vi "FT10_Log Tester Write TDMS.vi"(6 "Time in":timestamp, 8 "error in (no error)":errorcluster, 9 "Measurements in":T1, 10 "Waveform in":waveform(dbl), 11 "Refnum in":refnum<k34>) -> (0 "error out":errorcluster, 3 "Refnum out":refnum<k34>)   [LabVIEW 2015]
uses:
  <vilib>/Waveform/WDTOps.llb/WDT Number of Waveform Samples DBL.vi
  <vilib>/Waveform/WDTOps.llb/WDT Get Waveform Time Array DBL.vi
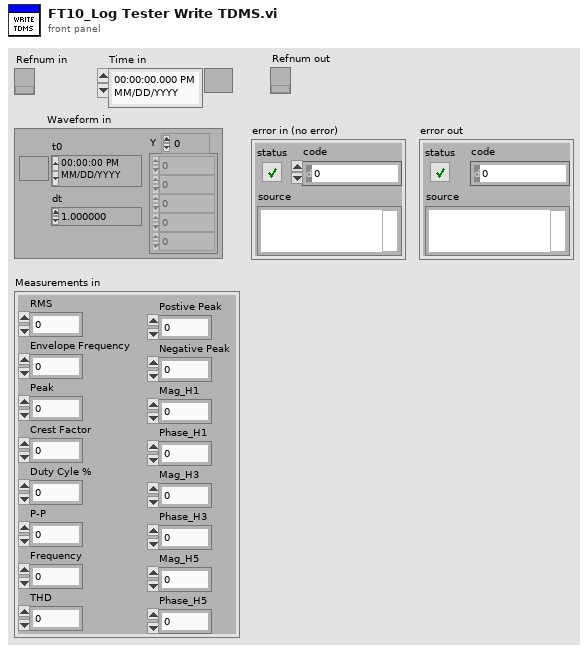
[diagram p1: front panel]
types:
  T1 = cluster{"RMS":dbl, "Envelope Frequency":dbl, "Peak":dbl, "Crest Factor":dbl, "Duty Cyle %":dbl, "P-P":dbl, "Frequency":dbl, "THD":dbl, "Postive Peak":dbl, "Negative Peak":dbl, "Mag_H1":dbl, "Phase_H1":dbl, "Mag_H3":dbl, "Phase_H3":dbl, "Mag_H5":dbl, "Phase_H5":dbl}
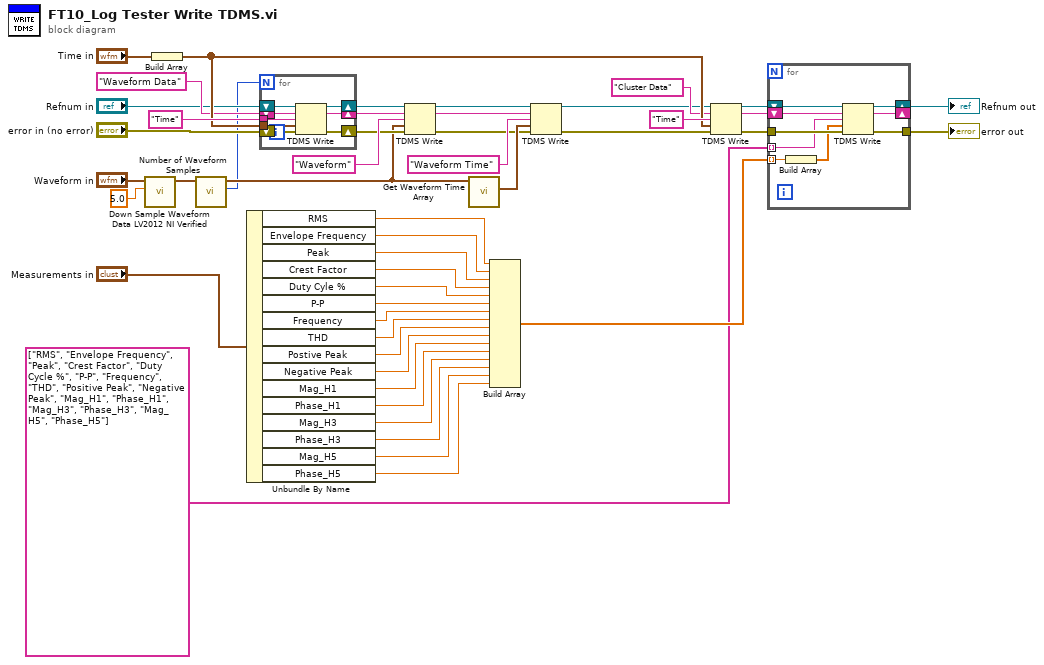
[diagram p0: block diagram]
diagram:
  n1 = call "Down Sample Waveform Data LV2012 NI Verified.vi"("Desired Sampling Rate"=5.0, "Waveform in"="Waveform in") -> ("Waveform out"=w2:waveform(dbl))  [unwired: 8 in, 1 out]
  n2 = Build Array("Time in") -> (w21:timestamp[])
  n3 = call-poly <vilib>:"Number of Waveform Samples.vi"("waveform in"=w2) -> ("number of samples"=w4:i32, "waveform out"=w5:waveform(dbl))  [unwired: 8 in, 1 out]
  n4 = Unbundle By Name("Measurements in") -> ("RMS"=w40:dbl, "Envelope Frequency"=w39:dbl, "Peak"=w38:dbl, "Crest Factor"=w37:dbl, "Duty Cyle %"=w36:dbl, "P-P"=w35:dbl, "Frequency"=w34:dbl, "THD"=w33:dbl, "Postive Peak"=w32:dbl, "Negative Peak"=w31:dbl, "Mag_H1"=w30:dbl, "Phase_H1"=w29:dbl, "Mag_H3"=w28:dbl, "Phase_H3"=w27:dbl, "Mag_H5"=w26:dbl, "Phase_H5"=w25:dbl)
  n5 = for {
    N: w4 -> [_]
    tunnel: "Time" ("channel name(s) in (Untitled)") -> [w56]
    tunnel: w21 -> [w55]
    shift-right: [w49] -> w8
    shift-left: "Waveform Data" ("group name in (Untitled)") -> [w54]
    shift-right: [w50] -> w9
    shift-left: "Refnum in" -> [w53]
    shift-right: [w51] -> w10
    shift-left: "error in (no error)" -> [w52]
    n6 = TDMS Write(0:w53, 5:w54, 7:w56, 9:w55, 11:w52) -> (4:w50:refnum<k34>, 6:w49:string, 15:w51:errorcluster)  [unwired: 1 in, 1 out]
  }
  n7 = TDMS Write(0:w9, 5:w8, 7:"Waveform" ("channel name(s) in (Untitled)"), 9:w5, 11:w10) -> (4:w45:refnum<k34>, 6:w14:string, 15:w46:errorcluster)  [unwired: 1 in, 1 out]
  n8 = call-poly <vilib>:"Get Waveform Time Array.vi"("waveform in"=w5) -> ("X array"=w47:timestamp[])  [unwired: 9 in, 1 out]
  n9 = Build Array(w40, w39, w38, w37, w36, w35, w34, w33, w32, w31, w30, w29, w28, w27, w26, w25) -> (w24:dbl[])
  n10 = TDMS Write(0:w45, 5:w14, 7:"Waveform Time" ("channel name(s) in (Untitled)"), 9:w47, 11:w46) -> (4:w7:refnum<k34>, 15:w6:errorcluster)  [unwired: 1 in, 2 out]
  n11 = TDMS Write(0:w7, 5:"Cluster Data" ("group name in (Untitled)"), 7:"Time" ("channel name(s) in (Untitled)"), 9:w21, 11:w6) -> (4:w19:refnum<k34>, 6:w18:string, 15:w17:errorcluster)  [unwired: 1 in, 1 out]
  n12 = for {
    shift-right: [w64] -> w16
    shift-left: w19 -> [w65]
    shift-right: [w62] -> _
    shift-left: w18 -> [w63]
    tunnel: w17 -> [w61]
    tunnel: [w60] -> w15
    tunnel: w24 -> [w59] mode=indexing
    tunnel: string[] ["RMS", "Envelope Frequency", "Peak", "Crest Factor", "Duty Cycle %", "P-P", "Frequency", "THD", "Positive Peak", "Negative Peak", "Mag_H1", "Phase_H1", "Mag_H3", "Phase_H3", "Mag_H5", "Phase_H5"] ("channel name(s) in (Untitled)") -> [w57] mode=indexing
    n13 = Build Array(w59) -> (w58:dbl[])
    n14 = TDMS Write(0:w65, 5:w63, 7:w57, 9:w58, 11:w61) -> (4:w64:refnum<k34>, 6:w62:string, 15:w60:errorcluster)  [unwired: 1 in, 1 out]
  }
  "error out" <- w15
  "Refnum out" <- w16
